vi "cmc-coin_flipper.vi"() -> ()   [LabVIEW 2010]
panel:
  out "Number of Updates":u32
  out "Elapsed Time (sec)":dbl
  out "Number of Flips":u32
  in  "stop":bool
  out "Tails":u64(slide) scale=0.0..473578644.0
  out "Heads":u64(slide) scale=0.0..473578644.0
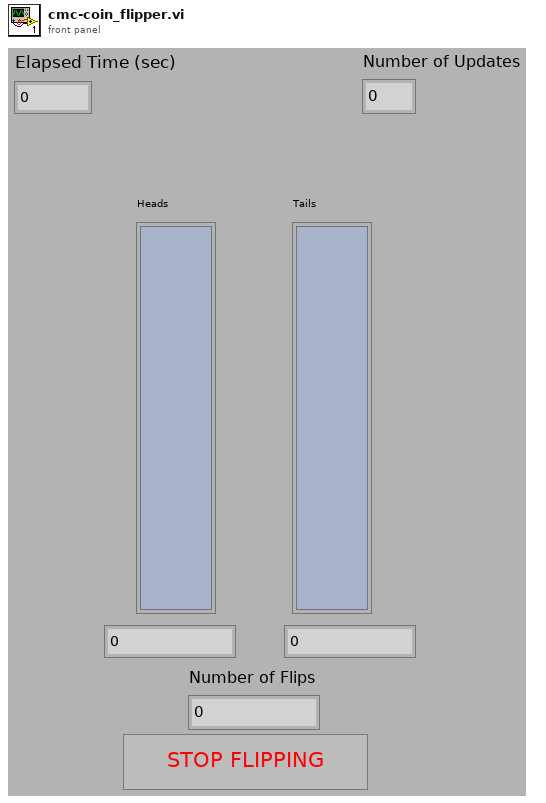
[diagram p1: front panel]
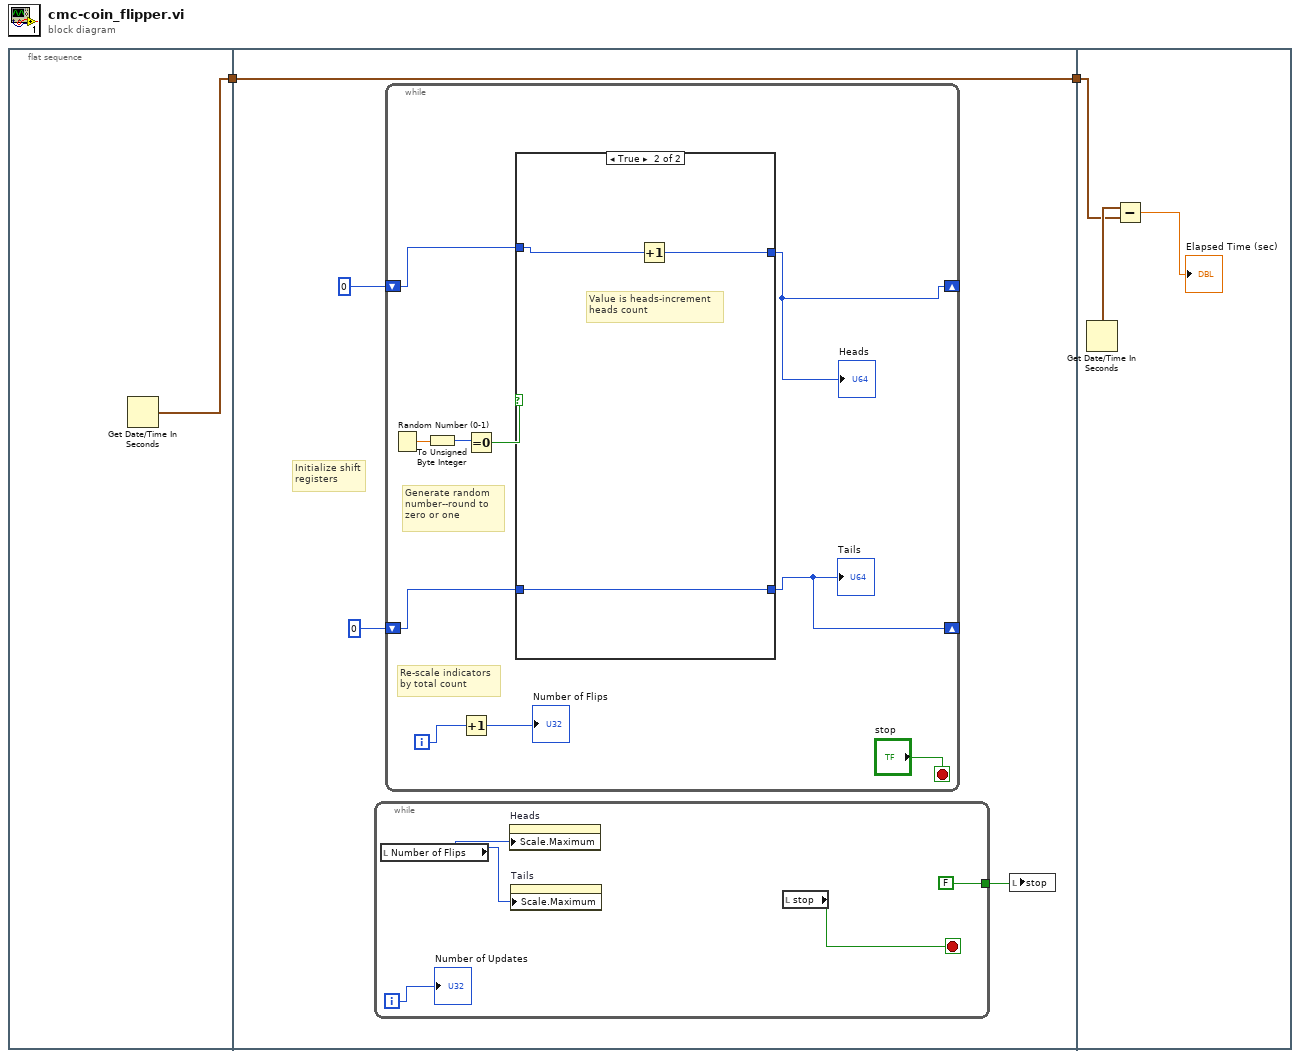
[diagram p0: block diagram]
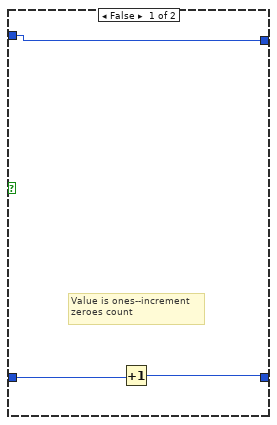
[diagram p2: hidden frame]
diagram:
  n1 = flat-sequence {
    tunnel: [w3] -> w2
    tunnel: w2 -> [w5]
    tunnel: [w5] -> w1
    tunnel: w1 -> [w28]
    frame #0 {
      n2 = Get Date/Time In Seconds() -> (seconds since 1Jan1904=w3:timestamp)
    }
    frame #1 {
      # "Initialize shift\nregisters"
      n3 = while {
        tunnel: [FALSE] -> w4
        i -> [w10]
        stop <- w9 stop-if-true
        n4 = local read "Number of Flips"() -> (w11:u32)
        n5 = property on="Heads" class="Slide (strict)"("Scale.Maximum"=w11) -> ()  [unwired: 2 in, 2 out]
        n6 = property on="Tails" class="Slide (strict)"("Scale.Maximum"=w11) -> ()  [unwired: 2 in, 2 out]
        n7 = local read "stop"() -> (w9:bool)
        "Number of Updates" <- w10
      }
      n8 = while {
        shift-right: [w15] -> _
        shift-left: 0 -> [w21]
        shift-right: [w14] -> _
        shift-left: 0 -> [w20]
        i -> [w13]
        stop <- "stop" stop-if-true
        # "Re-scale indicators\nby total count"
        # "Generate random\nnumber--round to\nzero or one"
        n9 = Random Number (0-1)() -> (number: 0 to 1=w19:dbl)
        n10 = To Unsigned Byte Integer(number=w19) -> (unsigned 8bit integer=w18:u8)
        n11 = Increment(x=w13) -> (x+1=→"Number of Flips":i32)
        n12 = Equal To 0?(x=w18) -> (x = 0?=w17:bool)
        n13 = case shown="True" w17 {
          tunnel: w21 -> [w24 w27]
          tunnel: w20 -> [w23 w25]
          tunnel: [w24 w26] -> w15
          tunnel: [w22 w25] -> w14
          frame False {
            # "Value is ones--increment\nzeroes count"
            n14 = Increment(x=w23) -> (x+1=w22:i32)
          }
          frame True {
            # "Value is heads-increment\nheads count"
            n15 = Increment(x=w27) -> (x+1=w26:i32)
          }
        }
        "Tails" <- w14
        "Heads" <- w15
      }
      n16 = local write "stop"(w4) -> ()
    }
    frame #2 {
      n17 = Get Date/Time In Seconds() -> (seconds since 1Jan1904=w29:timestamp)
      n18 = Subtract(x=w29, y=w28) -> (x-y=→"Elapsed Time (sec)":dbl)
    }
  }
